vi "isReporting.vi"(8 "error in (no error)":errorcluster, 11 "Test Report in":refnum<class "Test Report.lvclass">) -> (0 "error out":errorcluster, 2 "Exporting?":bool, 3 "Test Report out":refnum<class "Test Report.lvclass">)   [LabVIEW 2013, in "Caraya.lvlib" / "Test Report.lvclass"]
uses:
  Test Report.lvclass
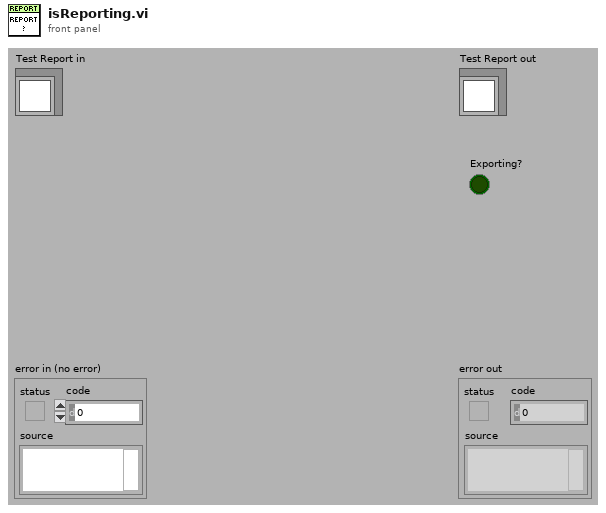
[diagram p1: front panel]
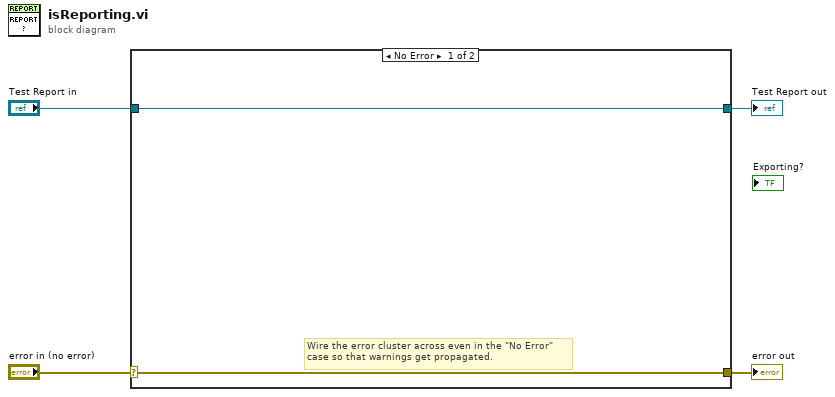
[diagram p0: block diagram]
diagram:
  n1 = case shown="No Error" "error in (no error)" {
    selector: "error in (no error)" -> [w5 w8]
    tunnel: [w5 w8] -> w3
    tunnel: [w6 w7] -> w1
    tunnel: "Test Report in" -> [w6 w7]
    frame No Error {
      # "Wire the error cluster across even in the \"No Error\"\ncase so that warnings get propagated."
    }
    frame Error {
    }
  }
  "error out" <- w3
  "Test Report out" <- w1
